vi "Koheras_Communication.vi"(3 "Error in":errorcluster, 4 "Answer length":u32, 5 "Command":string, 6 "VISA resource name in":refnum<visa-resource-name>) -> (0 "Error out":errorcluster, 1 "Returns":string, 2 "VISA resource name out":refnum<visa-resource-name>)   [LabVIEW 2009]
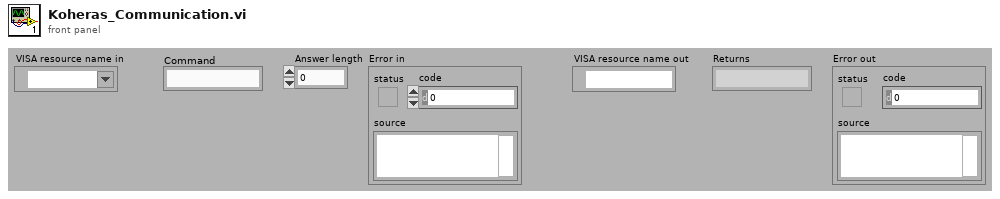
[diagram p1: front panel]
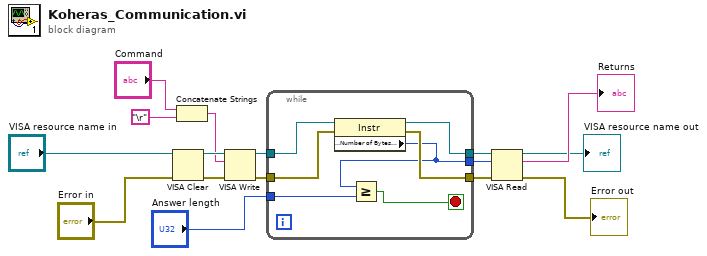
[diagram p0: block diagram]
diagram:
  n1 = VISA Clear(VISA resource name="VISA resource name in", error in (no error)="Error in") -> (VISA resource name out=w8:refnum<visa-resource-name>, error out=w7:errorcluster)
  n2 = Concatenate Strings("Command", "\r") -> (w5:string)
  n3 = VISA Write(VISA resource name=w8, write buffer=w5, error in (no error)=w7) -> (VISA resource name out=w9:refnum<visa-resource-name>, error out=w10:errorcluster)  [unwired: 1 out]
  n4 = while {
    tunnel: w9 -> [w23]
    tunnel: w10 -> [w22]
    tunnel: [w21] -> w11
    tunnel: [w20] -> w12
    tunnel: [w18] -> w13
    tunnel: "Answer length" -> [w17]
    stop <- w19 stop-if-true
    n5 = property class="Instr"(reference=w23, error in=w22) -> (reference out=w20:refnum<visa-resource-name>, error out=w21:errorcluster, "Serial Settings:Number of Bytes at Serial Port"=w18:u32)
    n6 = Greater Or Equal?(x=w18, y=w17) -> (x >= y?=w19:bool)
  }
  n7 = VISA Read(VISA resource name=w12, byte count=w13, error in (no error)=w11) -> (VISA resource name out=→"VISA resource name out":refnum<visa-resource-name>, read buffer=→"Returns":string, error out=→"Error out":errorcluster)  [unwired: 1 out]
